vi "Display_Main.vi"(8 "error in":errorcluster, 11 "QRD":T1) -> (0 "error out":errorcluster)   [LabVIEW 2025]
uses:
  Controls/Queues-Refs-Data.ctl
  Builds/Queue Wrappers.lvlibp/Q Packet.ctl
  Controls/Local Data_Display.ctl
  Controls/Acquisition Packet.ctl
  Builds/Queue Wrappers.lvlibp
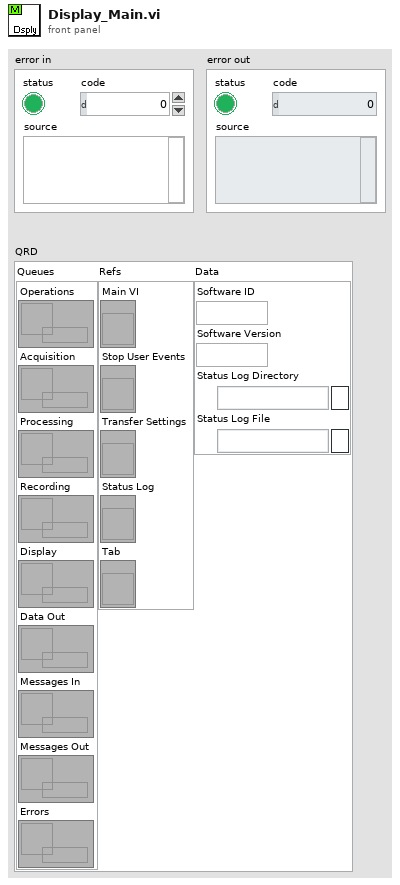
[diagram p1: front panel]
types:
  T1 = typedef "Queues-Refs-Data.ctl" = cluster{"Queues":cluster{"Operations":refnum<queue>, "Acquisition":refnum<queue>, "Processing":refnum<queue>, "Recording":refnum<queue>, "Display":refnum<queue>, "Data Out":refnum<queue>, "Messages In":refnum<queue>, "Messages Out":refnum<queue>, "Errors":refnum<queue>}, "Refs":cluster{"Main VI":refnum<vi>, "Stop User Events":refnum<vi>, "Transfer Settings":refnum<vi>, "Status Log":refnum<vi>, "Tab":refnum<vi>}, "Data":cluster{"Software ID":string, "Software Version":string, "Status Log Directory":path, "Status Log File":path}}
  T2 = typedef "Local Data_Display.ctl" = cluster{"Loop ID":string, "Refresh Rate":dbl, "Last Update":dbl, "Acqusition Buffer":T3[]}
  T3 = typedef "Acquisition Packet.ctl" = cluster{"Time Stamp":timestamp, "Raw Data":cluster{"String":string, "Numeric":dbl, "Boolean":bool}, "Derived Data":cluster{"String":string, "Numeric":dbl, "Boolean":bool}}
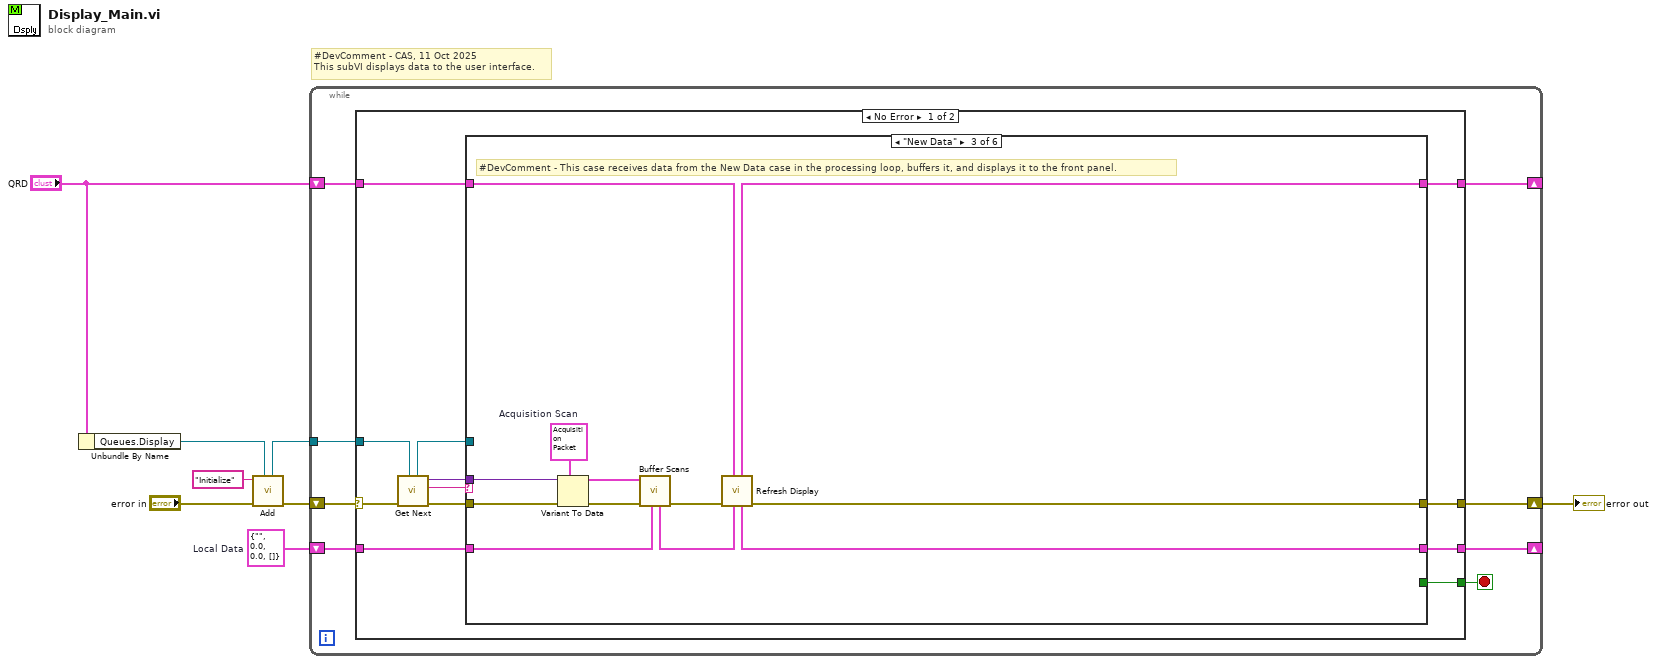
[diagram p0: block diagram]
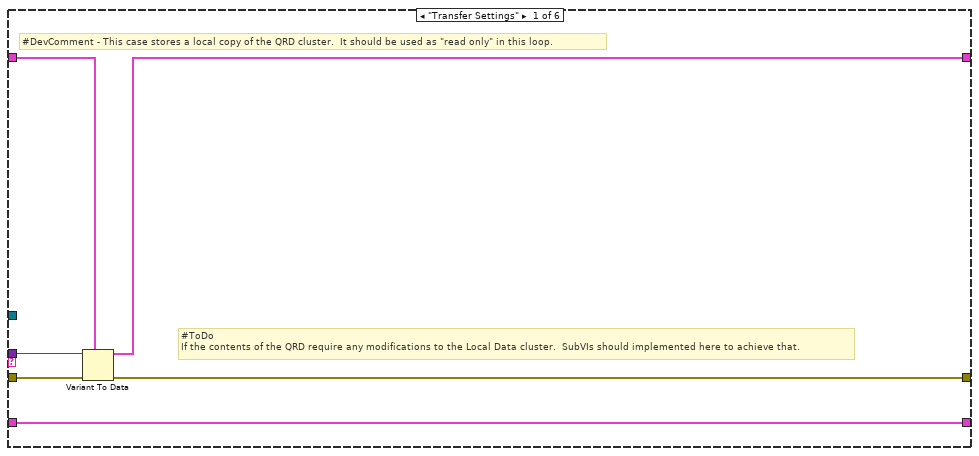
[diagram p2: hidden frame]
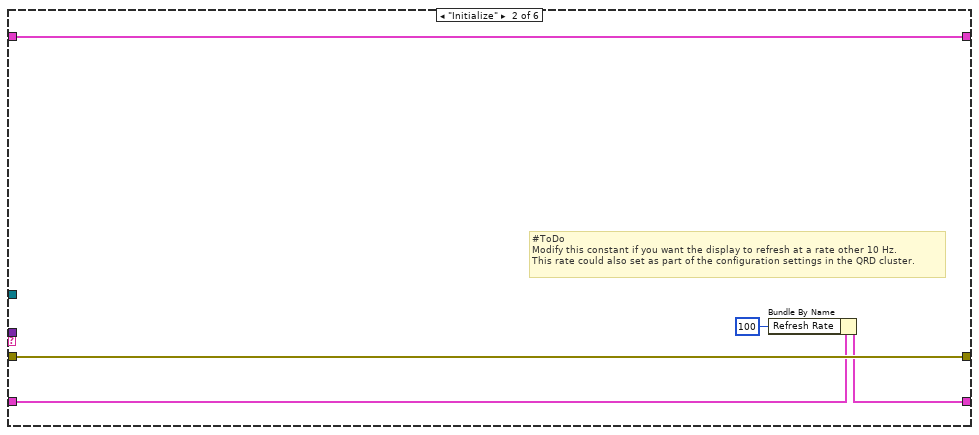
[diagram p3: hidden frame]
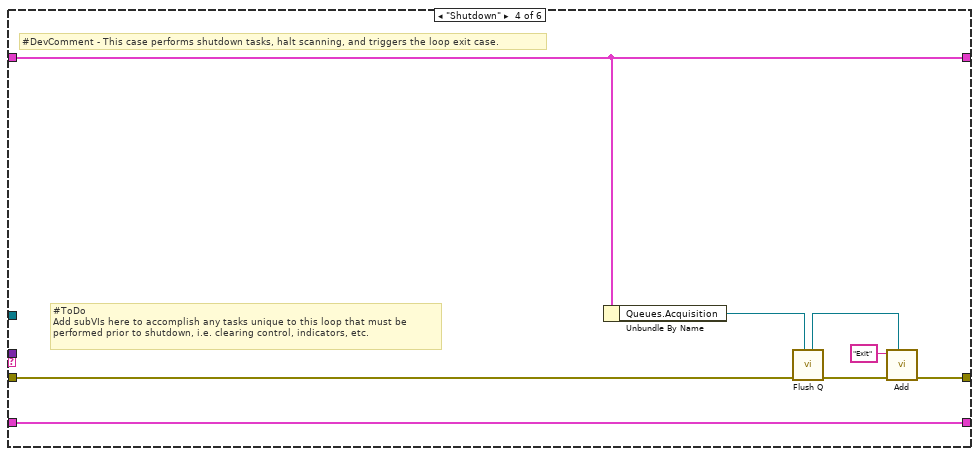
[diagram p4: hidden frame]
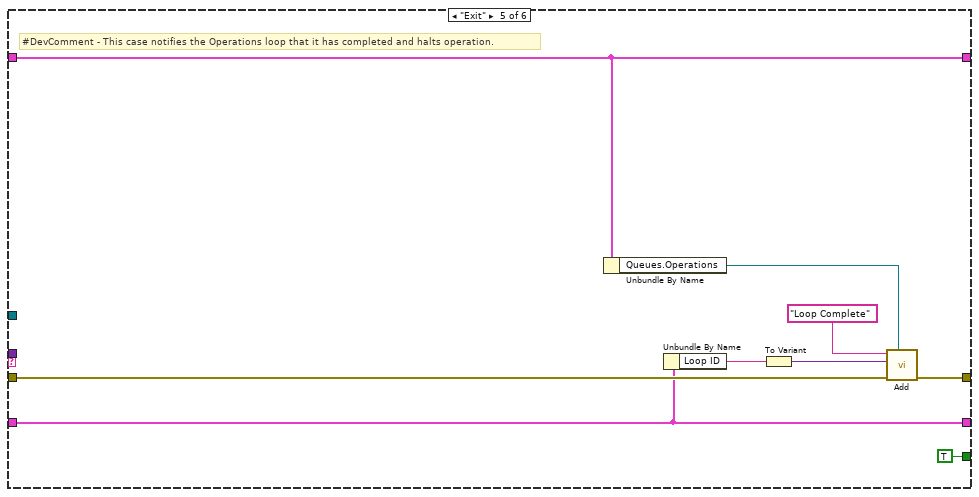
[diagram p5: hidden frame]
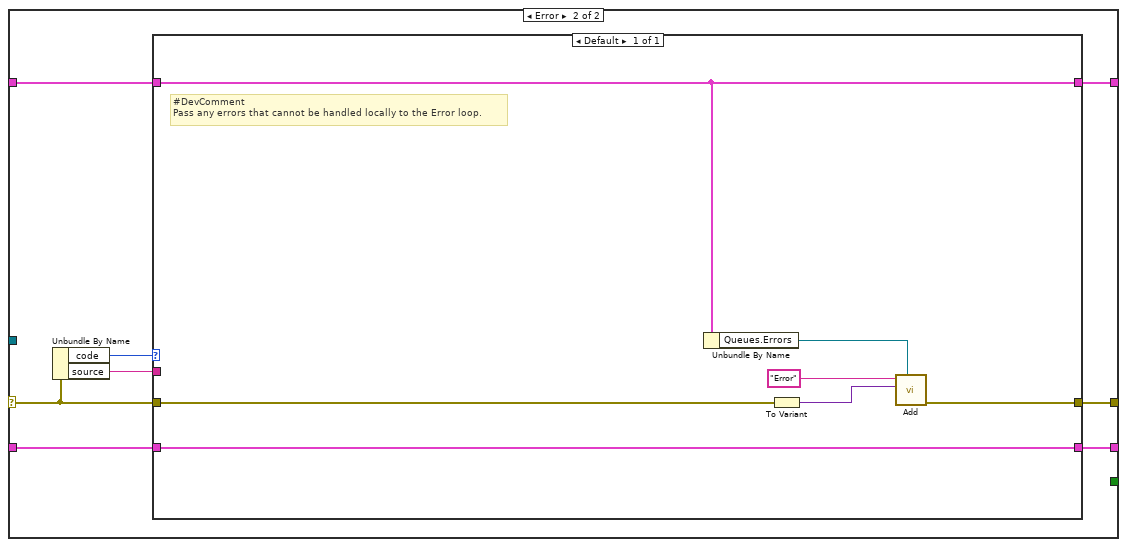
[diagram p7: hidden frame]
diagram:
  w6 = T2 {"Loop ID"="", "Refresh Rate"=0.0, "Last Update"=0.0, "Acqusition Buffer"=[]}  # Local Data
  # "#DevComment - CAS, 11 Oct 2025\nThis subVI displays data to the user interface."
  n1 = Unbundle By Name("QRD") -> ("Queues.Display"=w3:refnum<queue>)
  n2 = call "Add.vi"("Q Ref In"=w3, "error in"="error in", "Packet ID"="Initialize") -> ("error out"=w4:errorcluster, "Q Ref Out"=w2:refnum<queue>)  [unwired: 5 in, 2 out]
  n3 = while {
    shift-right: [w15] -> _
    shift-left: "QRD" -> [w16]
    shift-right: [w13] -> w8
    shift-left: w4 -> [w14]
    tunnel: w2 -> [w12]
    shift-right: [w9] -> _
    shift-left: w6 -> [w11]
    stop <- w10 stop-if-true
    n4 = case shown="No Error" w14 {
      selector: w14 -> [w28 w76]
      tunnel: w16 -> [w25 w73]
      tunnel: [w26 w74] -> w15
      tunnel: [w23 w75] -> w13
      tunnel: w12 -> [w27 _]
      tunnel: w11 -> [w19 w77]
      tunnel: [w18 w72] -> w9
      tunnel: [w17 _] -> w10
      frame No Error {
        n5 = call "Get Next.vi"("Q Ref In"=w27, "error in"=w28) -> ("error out"=w24:errorcluster, "Packet ID"=w20:string, "Payload"=w21:variant, "Q Ref Out"=w22:refnum<queue>)  [unwired: 6 in]
        n6 = case shown="\"New Data\"" w20 {
          tunnel: [w30 w39 w41 w59 w68 w71] -> w26
          tunnel: w25 -> [w32 w39 w40 w59 w68 w71]
          tunnel: w24 -> [w34 w38 w51 w56 w65 w70]
          tunnel: [w31 w38 w46 w58 w67 w70] -> w23
          tunnel: w22 -> [_ _ _ _ _ _]
          tunnel: w21 -> [w33 _ w50 _ _ _]
          tunnel: w19 -> [w29 w36 w43 w52 w63 w69]
          tunnel: [w29 w37 w44 w52 w63 w69] -> w18
          tunnel: [_ _ _ _ TRUE _] -> w17
          frame "Transfer Settings" {
            # "#ToDo\nIf the contents of the QRD require any modifications to the Local Data cluster.  SubVIs should implemented here to achieve that."
            # "#DevComment - This case stores a local copy of the QRD cluster.  It should be used as \"read only\" in this loop."
            n7 = Variant To Data(error in=w34, type=w32, Variant=w33) -> (data=w30:T1, error out=w31:errorcluster)
          }
          frame "Initialize" {
            # "#ToDo\nModify this constant if you want the display to refresh at a rate other 10 Hz.\nThis rate could also set as part of the configuration settings in the QRD cluster."
            n8 = Bundle By Name(cluster=w36, "Refresh Rate"=100) -> (w37:T2)
          }
          frame "New Data" {
            w49 = T3 {"Time Stamp"=timestamp(0 s since 1904-01-01), "Raw Data"={"String"="", "Numeric"=0.0, "Boolean"=FALSE}, "Derived Data"={"String"="", "Numeric"=0.0, "Boolean"=FALSE}}  # Acquisition Scan
            # "#DevComment - This case receives data from the New Data case in the processing loop, buffers it, and displays it to the front panel."
            n9 = Variant To Data(error in=w51, type=w49, Variant=w50) -> (data=w42:T3, error out=w47:errorcluster)
            n10 = call "Buffer Scans.vi"("Local Data"=w43, "error in"=w47, "Acquisition Scan"=w42) -> ("error out"=w48:errorcluster, "Local Data Out"=w45:T2)  [unwired: 7 in]
            n11 = call "Refresh Display.vi"("Local Data"=w45, "QRD"=w40, "error in"=w48) -> ("error out"=w46:errorcluster, "Local Data Out"=w44:T2, "QRD Out"=w41:T1)  [unwired: 6 in]
          }
          frame "Shutdown" {
            # "#ToDo\nAdd subVIs here to accomplish any tasks unique to this loop that must be\nperformed prior to shutdown, i.e. clearing control, indicators, etc."
            # "#DevComment - This case performs shutdown tasks, halt scanning, and triggers the loop exit case."
            n12 = Unbundle By Name(w59) -> ("Queues.Acquisition"=w54:refnum<queue>)
            n13 = call "Flush Q.vi"("Q Ref In"=w54, "error in"=w56) -> ("error out"=w55:errorcluster, "Q Ref Out"=w53:refnum<queue>)  [unwired: 8 in]
            n14 = call "Add.vi"("Q Ref In"=w53, "error in"=w55, "Packet ID"="Exit") -> ("error out"=w58:errorcluster)  [unwired: 5 in, 3 out]
          }
          frame "Exit" {
            # "#DevComment - This case notifies the Operations loop that it has completed and halts operation."
            n15 = Unbundle By Name(w68) -> ("Queues.Operations"=w64:refnum<queue>)
            n16 = Unbundle By Name(w63) -> ("Loop ID"=w62:string)
            n17 = To Variant(anything=w62) -> (Variant=w61:variant)
            n18 = call "Add.vi"("Q Ref In"=w64, "error in"=w65, "Payload"=w61, "Packet ID"="Loop Complete") -> ("error out"=w67:errorcluster)  [unwired: 4 in, 3 out]
          }
          frame Default {
          }
        }
      }
      frame Error {
        n19 = Unbundle By Name(w76) -> ("code"=w79:i32, "source"=w78:string)
        n20 = case shown="Default" w79 {
          tunnel: w78 -> [_]
          tunnel: w77 -> [w86]
          tunnel: [w86] -> w72
          tunnel: w76 -> [w81]
          tunnel: [w83] -> w75
          tunnel: [w82] -> w74
          tunnel: w73 -> [w82]
          frame Default {
            # "#DevComment\nPass any errors that cannot be handled locally to the Error loop."
            n21 = Unbundle By Name(w82) -> ("Queues.Errors"=w84:refnum<queue>)
            n22 = To Variant(anything=w81) -> (Variant=w80:variant)
            n23 = call "Add.vi"("Q Ref In"=w84, "Payload"=w80, "Packet ID"="Error") -> ("error out"=w83:errorcluster)  [unwired: 5 in, 3 out]
          }
        }
      }
    }
  }
  "error out" <- w8
